vi "SECoP-addStatusParameter.vi"(6 "description":string, 7 "states":T1[](array[typedef])=[{"value"=100, "name"="IDLE"}, {"value"=300, "name"="BUSY"}] {"value" max=999 step=1 format="%03.0f"}, 8 "error in (no error)":errorcluster, 10 "parameter name":string="status", 11 "DLL path (in)":T2) -> (0 "error out":errorcluster, 3 "DLL path (out)":T2)   [LabVIEW 2023, in "SECoP.lvlib"]
doc: "Call <b>\"SECoP-addStatusParameter.vi\"</b> to create a read only SECoP status parameter with predefined states inside the last created SECoP module.\n\n<b>DLL path</b> input and output of cluster from \"SECoP-Initialize.vi\"\noptional <b>parameter name</b> name of parameter (default: status)\n<b>states</b> list of states (see SECoP specification)\n<b>description</b> human readable description of this parameter"
uses:
  SECoP.lvlib
  SECoP-libraries.ctl
  SECoP-statusValue.ctl
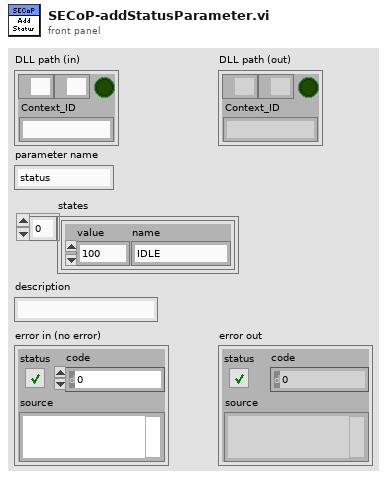
[diagram p1: front panel]
types:
  T1 = typedef "SECoP.lvlib/SECoP-statusValue.ctl" = cluster{"value":u64, "name":string}
  T2 = typedef "SECoP.lvlib/SECoP-libraries.ctl" = cluster{"serverDLL":path, "variantDLL":path, "cleanup_mode":bool, "Context_ID":string}
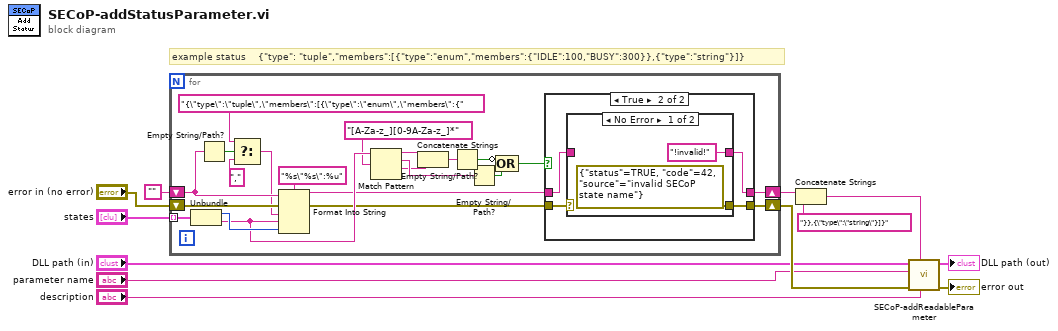
[diagram p0: block diagram]
diagram:
  # "example status    {\"type\": \"tuple\",\"members\":[{\"type\":\"enum\",\"members\":{\"IDLE\":100,\"BUSY\":300}},{\"type\":\"string\"}]}"
  n1 = for {
    tunnel: "states" -> [w33] mode=indexing
    shift-right: [w13] -> w7
    shift-left: "" -> [w26]
    shift-right: [w15] -> w12
    shift-left: "error in (no error)" -> [w28]
    n2 = Unbundle(w33) -> ("value"=w27:u64, "name"=w24:string)
    n3 = Empty String/Path?(string/path=w26) -> (empty?=w32:bool)
    n4 = Select(t="{\"type\":\"tuple\",\"members\":[{\"type\":\"enum\",\"members\":{", s=w32, f=",") -> (s? t:f=w25:string)
    n5 = Format Into String(format string="%s\"%s\":%u", initial string=w26, error in=w28, w25, w24, w27) -> (resulting string=w14:string, error out=w17:errorcluster)
    n6 = Match Pattern(string=w24, regular expression="[A-Za-z_][0-9A-Za-z_]*") -> (before substring=w22:string, match substring=w34:string, after substring=w21:string)  [unwired: 1 in, 1 out]
    n7 = Concatenate Strings(w22, w21) -> (w20:string)
    n8 = Empty String/Path?(string/path=w20) -> (empty?=w19:bool)
    n9 = Empty String/Path?(string/path=w34) -> (empty?=w18:bool)
    n10 = Compound Arithmetic op=OR(invert w19, w18) -> (w16:bool)
    n11 = case shown="True" w16 {
      tunnel: w17 -> [w36 w40]
      tunnel: [w36 w37] -> w15
      tunnel: w14 -> [w35 w39]
      tunnel: [w35 w38] -> w13
      frame False {
      }
      frame True {
        n12 = case shown="No Error" w40 {
          selector: w40 -> [_ w44]
          tunnel: [errorcluster {"status"=TRUE, "code"=42, "source"="invalid SECoP state name"} ("error IO") w44] -> w37
          tunnel: w39 -> [_ w43]
          tunnel: ["!invalid!" w43] -> w38
          frame No Error {
          }
          frame Error {
          }
        }
      }
    }
  }
  n13 = Concatenate Strings(w7, "}},{\"type\":\"string\"}]}" ("string")) -> (w4:string)
  n14 = call "SECoP-addReadableParameter.vi"("description"="description", "datainfo"=w4, "error in (no error)"=w12, "parameter name"="parameter name", "DLL path (in)"="DLL path (in)") -> ("error out"=→"error out":errorcluster, "DLL path (out)"=→"DLL path (out)":T2)  [unwired: 5 in]
